vi "SiggenRfOff.vi"(2 "error in (no error)":errorcluster) -> (0 "error out":errorcluster)   [LabVIEW 2009]
doc: "Turn OFF siggen RF."
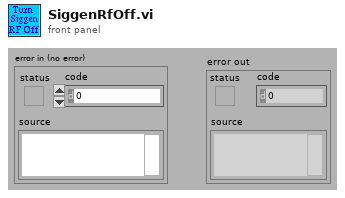
[diagram p1: front panel]
types:
  T1 = enum16{"N1911A", "Siggen", "34980a", "E4418B", "Rvp8"}
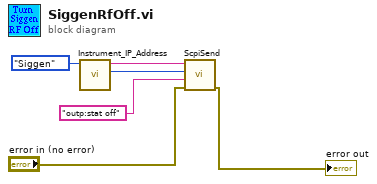
[diagram p0: block diagram]
diagram:
  n1 = call "Instrument_IP_Address.vi"("Instrument"=T1."Siggen") -> ("Port"=w1:u16, "IP Address"=w2:string)  [unwired: 9 in]
  n2 = call "ScpiSend.vi"("error in (no error)"="error in (no error)", "Command"="outp:stat off" ("format string"), "TCP port"=w1, "IP Address"=w2) -> ("error out"=→"error out":errorcluster)  [unwired: 7 in]
